vi "AppLauncher.vi"() -> ()   [LabVIEW 2016, in "Instrument.SR7270.lvclass"]
uses:
  Instrument.SR7270.lvclass
  <vilib>/JKI/JKI SMO/SMO/SMO.lvclass
  <vilib>/JKI/JKI SMO/SMO/Typedefs/SMOState --Enum.ctl
  <vilib>/JKI/JKI SMO/SMO.UI/SMO.UI.lvclass
  SR7270 UI/SR7270 UI.lvclass
  C:/user/patrick/hg/levylab_inst/lvsrc/SMOs/Instrument/Instrument.lvclass
  C:/Program Files (x86)/National Instruments/LabVIEW 2016/vi.lib/JKI/JKI SMO/SMO/SMO.lvclass
  C:/Program Files (x86)/National Instruments/LabVIEW 2016/vi.lib/JKI/JKI SMO/SMO.UI/SMO.UI.lvclass
  <vilib>/Utility/sysdir.llb/System Directory Type.ctl
panel:
  out "UI SMO State":T1
  out "SMO State":T1
  out "error out":errorcluster
  in  "Stop":bool
  # "Instrument.SR7270 SMO Launcher"
  # "For instructions on how to use the JKI State Machine Objects, examples and video tutorials, visit:\nhttp://jki.net/state-machine-objects/\n\nJKI State Machine Objects™\nhttp://jki.net/state-machine-objects/\nCopyright (C) 2005-2015, JKI <info@jki.net>\nALL RIGHTS RESERVED"
  # "Starting SR7270 SMO..."
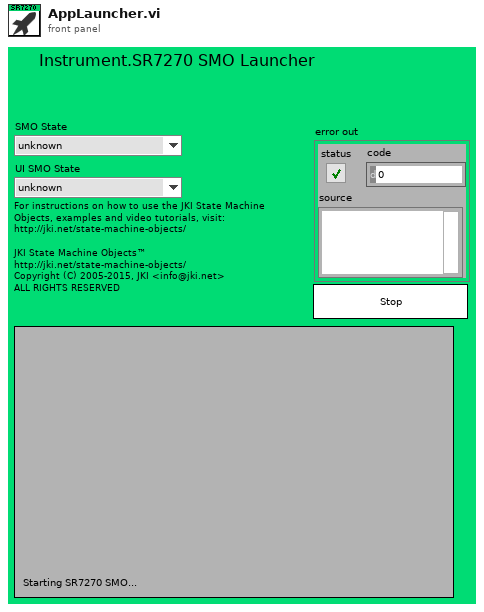
[diagram p1: front panel]
types:
  T1 = typedef "SMO.lvclass/SMOState --Enum.ctl" = enum16{"unknown", "Created", "Started", "Stopped"}
  T2 = typedef "System Directory Type.ctl" = i32
  T3 = typedef "SMO.lvclass/Public Events.ctl" = cluster{"Error":refnum<user-event>, "State":refnum<user-event>, "Reserve State":refnum<user-event>}
  T4 = cluster{"Event Registration Refnum":refnum<event-registration>, "Event Registration Refnum":refnum<event-registration>}
  T5 = enum32{"Invalid", "Standard", "Closed", "Hidden", "Minimized", "Maximized"}
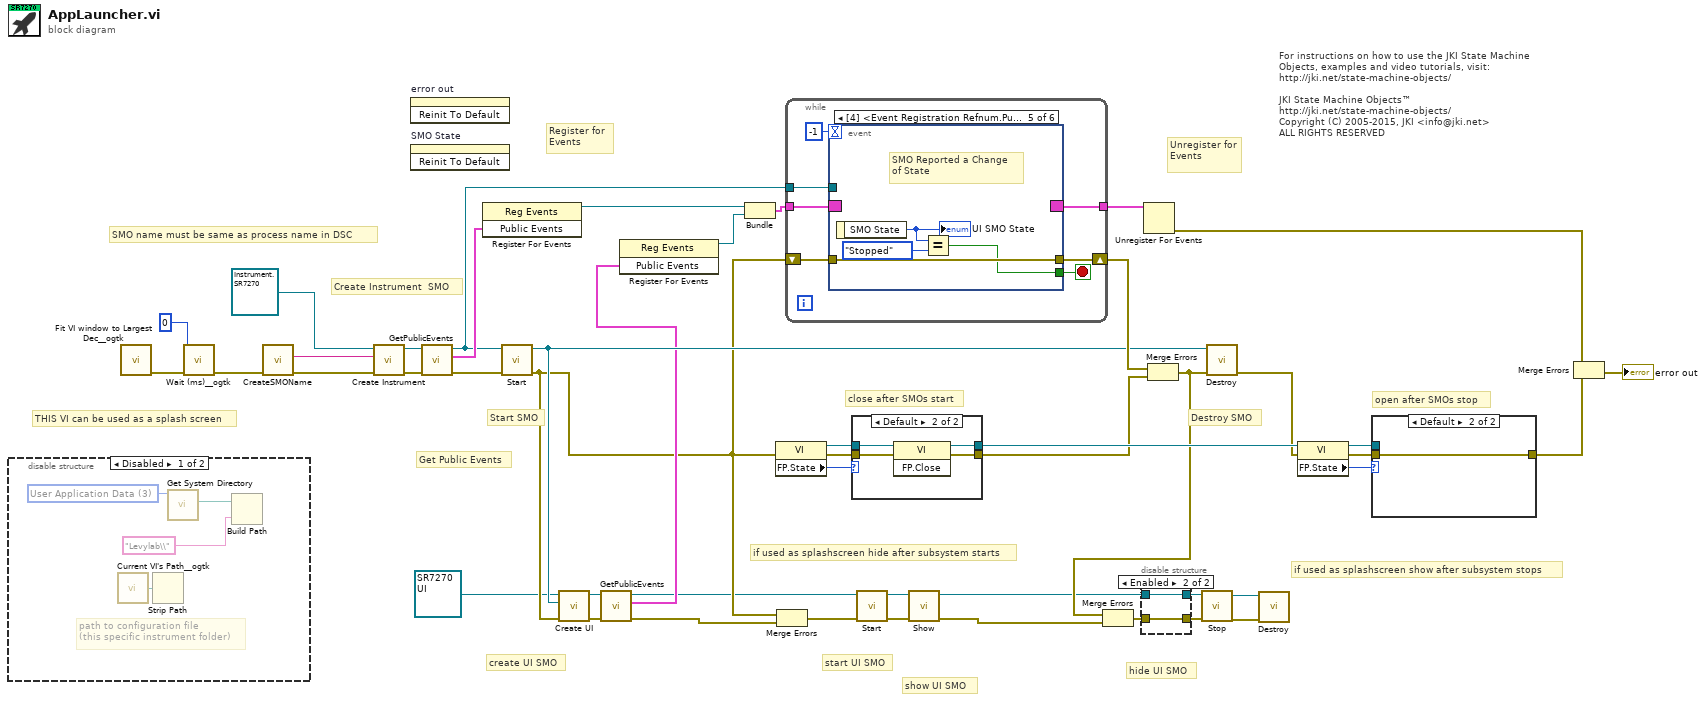
[diagram p0: block diagram]
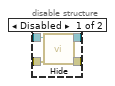
[diagram p3: hidden frame]
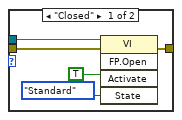
[diagram p4: hidden frame]
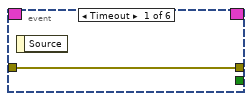
[diagram p6: hidden frame]
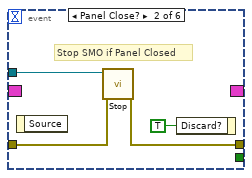
[diagram p7: hidden frame]
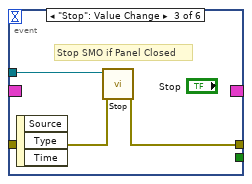
[diagram p8: hidden frame]
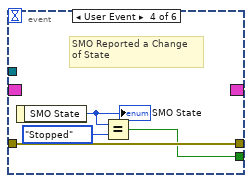
[diagram p9: hidden frame]
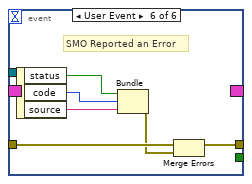
[diagram p10: hidden frame]
diagram:
  # "open after SMOs stop"
  # "close after SMOs start"
  # "hide UI SMO"
  # "show UI SMO"
  # "start UI SMO"
  # "create UI SMO"
  # "if used as splashscreen show after subsystem stops"
  # "if used as splashscreen hide after subsystem starts"
  # "THIS VI can be used as a splash screen"
  # "SMO name must be same as process name in DSC"
  # "Get Public Events"
  # "Start SMO"
  # "Destroy SMO"
  # "Create Instrument  SMO"
  # "Unregister for Events"
  # "Register for Events"
  # "For instructions on how to use the JKI State Machine Objects, examples and video tutorials, visit:\nhttp://jki.net/state-machine-objects/\n\nJKI State Machine Objects™\nhttp://jki.net/state-machine-objects/\nCopyright (C) 2005-2015, JKI <info@jki.net>\nALL RIGHTS RESERVED"
  n1 = disable-structure shown="Disabled" {
    frame Disabled {
      w50 = T2 3 items=["User Home"=0, "User Desktop"=1, "User Documents"=2, "User Application Data"=3, "User Preferences"=4, "User Temporary"=5, "Public Documents"=6, "Public Application Data"=7, "Public Preferences"=8, "Public Cache"=13, "System Core Libraries"=9, "System Installed Libraries"=10, "Application Files"=11, "Boot Volume Root"=12] ("system directory type")
      # "path to configuration file\n(this specific instrument folder)"
      n2 = call <userlib>:"Current VI's Path__ogtk.vi"() -> ("Current VI's Path (+ Relative)"=w51:path)  [unwired: 1 in]
      n3 = Strip Path(path=w51) -> ()  [unwired: 2 out]
      n4 = call <vilib>:"Get System Directory.vi"("system directory type"=w50) -> ("system directory"=w49:path)  [unwired: 10 in]
      n5 = Build Path(base path=w49, name or relative path="Levylab\\") -> ()  [unwired: 1 out]
    }
    frame Enabled {
    }
  }
  n6 = call <userlib>:"Fit VI window to Largest Dec__ogtk.vi"() -> ("error out"=w34:errorcluster)  [unwired: 6 in, 1 out]
  n7 = call <userlib>:"Wait (ms)__ogtk.vi"("error in (no error)"=w34, "milliseconds to wait"=u32 0) -> ("error out"=w3:errorcluster)  [unwired: 8 in, 1 out]
  n8 = call "CreateSMOName.vi"("error in (no error)"=w3) -> ("error out"=w1:errorcluster, "Name"=w2:string)  [unwired: 9 in]
  n9 = call-dynamic "Create Instrument.vi"("error in (no error)"=w1, "Subsystem Name"=w2, "Instrument in"=refnum<class "Instrument.SR7270.lvclass"> refnum ("Instrument.SR7270.lvclass")) -> ("error out"=w41:errorcluster, "Instrument out"=w42:refnum<class "Instrument.SR7270.lvclass">)  [unwired: 7 in]
  n10 = invoke on="error out" class="Clust (strict)" method="Reinit To Default"() -> ()  [unwired: 3 in, 3 out]
  n11 = invoke on="SMO State" class="Enum (strict)" method="Reinit To Default"() -> ()  [unwired: 3 in, 3 out]
  n12 = call <vilib>:"GetPublicEvents.vi"("error in (no error)"=w41, "SMO"=w42) -> ("error out"=w40:errorcluster, "Public Events"=w44:T3, "SMO out"=w43:refnum<class "Instrument.SR7270.lvclass">)  [unwired: 7 in]
  n13 = register-events(w44) -> (reference out=w33:refnum<event-registration>)  [unwired: 2 in, 1 out]
  n14 = call <vilib>:"Start.vi"("error in (no error)"=w40, "SMO"=w43) -> ("error out"=w26:errorcluster, "SMO out"=w31:refnum<class "Instrument.SR7270.lvclass">)  [unwired: 8 in]
  n15 = call "Create UI.vi"("error in (no error)"=w26, "Instrument in"=w31, "SR7270 UI in"=refnum<class "SR7270 UI.lvclass"> refnum ("SR7220 UI.lvclass")) -> ("error out"=w29:errorcluster, "SR7270 UI out"=w28:refnum<class "SR7270 UI.lvclass">)  [unwired: 7 in]
  n16 = call <vilib>:"GetPublicEvents.vi"("error in (no error)"=w29, "SMO"=w28) -> ("error out"=w20:errorcluster, "Public Events"=w27:T3, "SMO out"=w21:refnum<class "SR7270 UI.lvclass">)  [unwired: 7 in]
  n17 = register-events(w27) -> (reference out=w30:refnum<event-registration>)  [unwired: 2 in, 1 out]
  n18 = Bundle("Event Registration Refnum"=w33, "Event Registration Refnum"=w30) -> (w32:T4)  [unwired: 1 in]
  n19 = property class="VI"(error in=w26) -> (reference out=w9:refnum<vi>, error out=w10:errorcluster, "FP.State"=w8:T5)  [unwired: 1 in]
  n20 = Merge Errors(w26, w20) -> (w25:errorcluster)
  n21 = while {
    shift-right: [w57] -> w39
    shift-left: w26 -> [w56]
    tunnel: w32 -> [w55]
    tunnel: [w54] -> w47
    tunnel: w43 -> [w53]
    stop <- w58 stop-if-true
    n22 = event shown="[4] <Event Registration Refnum.Public Events.State>: User Event" {
      selector: w55 -> [_ _ _ _ _ _]
      dyn-events: [_ _ _ _ _ _] -> w54
      timeout: -1 -> [_ _ _ _ _ _]
      tunnel: [_ _ _ w67 w71 _] -> w58
      tunnel: w53 -> [_ w63 w66 _ _ _]
      tunnel: [w59 w62 w65 w70 w74 w78] -> w57
      tunnel: w56 -> [w59 w61 w64 w70 w74 w76]
      event Timeout {
        n23 = event-data() -> ()  [unwired: 1 in, 1 out]
      }
      event Panel Close? {
        # "Stop SMO if Panel Closed"
        n24 = event-data() -> ()  [unwired: 1 in, 1 out]
        n25 = call <vilib>:"Stop.vi"("error in (no error)"=w61, "SMO"=w63) -> ("error out"=w62:errorcluster)  [unwired: 8 in, 1 out]
        n26 = event-data("Discard?"=TRUE ("OK")) -> ()  [unwired: 1 in, 1 out]
      }
      event "Stop": Value Change {
        # "Stop SMO if Panel Closed"
        n27 = event-data() -> ()  [unwired: 1 in, 3 out]
        n28 = call <vilib>:"Stop.vi"("error in (no error)"=w64, "SMO"=w66) -> ("error out"=w65:errorcluster)  [unwired: 8 in, 1 out]
      }
      event User Event {
        # "SMO Reported a Change\nof State"
        n29 = event-data() -> ("SMO State"=w69:T1)  [unwired: 1 in]
        "SMO State" <- w69
        n30 = Equal?(x=w69, y=SMOState_--Enum."Stopped") -> (x = y?=w67:bool)
      }
      event User Event {
        # "SMO Reported a Change\nof State"
        n31 = event-data() -> ("SMO State"=w73:T1)  [unwired: 1 in]
        "UI SMO State" <- w73
        n32 = Equal?(x=w73, y=SMOState_--Enum."Stopped") -> (x = y?=w71:bool)
      }
      event User Event {
        # "SMO Reported an Error"
        n33 = event-data() -> ("status"=w77:bool, "code"=w80:i32, "source"=w79:string)  [unwired: 1 in]
        n34 = Bundle("status"=w77, "code"=w80, "source"=w79) -> (w75:errorcluster)  [unwired: 1 in]
        n35 = Merge Errors(w76, w75) -> (w78:errorcluster)
      }
    }
  }
  n36 = case shown="Default" w8 {
    tunnel: [w82 w86] -> w35
    tunnel: w10 -> [w82 w85]
    tunnel: w9 -> [w81 w84]
    tunnel: [w81 w83] -> w38
    frame "Invalid", "Closed" {
    }
    frame Default {
      n37 = invoke class="VI" method="FP.Close"(reference=w84, error in=w85) -> (reference out=w83:refnum<vi>, error out=w86:errorcluster)  [unwired: 1 in, 1 out]
    }
  }
  n38 = call <vilib>:"Start.vi"("error in (no error)"=w25, "SMO"=w21) -> ("error out"=w19:errorcluster, "SMO out"=w18:refnum<class "SR7270 UI.lvclass">)  [unwired: 8 in]
  n39 = call <vilib>:"Show.vi"("error in (no error)"=w19, "SMO.UI"=w18) -> ("error out"=w17:errorcluster, "SMO.UI out"=w13:refnum<class "SR7270 UI.lvclass">)  [unwired: 8 in]
  n40 = Unregister For Events(event registration refnum=w47) -> (error out=w46:errorcluster)  [unwired: 1 in]
  n41 = Merge Errors(w39, w35) -> (w22:errorcluster)
  n42 = Merge Errors(w22, w17) -> (w14:errorcluster)
  n43 = disable-structure shown="Enabled" {
    disable-tunnel: [w90 w91] -> w16
    disable-tunnel: [w89 w92] -> w15
    disable-tunnel: w14 -> [w88 w91]
    disable-tunnel: w13 -> [w87 w92]
    frame Disabled {
      n44 = call <vilib>:"Hide.vi"("error in (no error)"=w88, "SMO.UI"=w87) -> ("error out"=w90:errorcluster, "SMO.UI out"=w89:refnum<class "SR7270 UI.lvclass">)  [unwired: 8 in]
    }
    frame Enabled {
    }
  }
  n45 = call <vilib>:"Stop.vi"("error in (no error)"=w16, "SMO"=w15) -> ("error out"=w24:errorcluster, "SMO out"=w23:refnum<class "SR7270 UI.lvclass">)  [unwired: 8 in]
  n46 = call <vilib>:"Destroy.vi"("error in (no error)"=w22, "SMO"=w31) -> ("error out"=w37:errorcluster)  [unwired: 9 in]
  n47 = call <vilib>:"Destroy.vi"("error in (no error)"=w24, "SMO"=w23) -> ()  [unwired: 9 in, 1 out]
  n48 = property class="VI"(reference=w38, error in=w37) -> (reference out=w6:refnum<vi>, error out=w7:errorcluster, "FP.State"=w5:T5)
  n49 = case shown="Default" w5 {
    tunnel: [w95 w98] -> w36
    tunnel: w7 -> [w94 w98]
    tunnel: w6 -> [w93 _]
    frame "Closed" {
      n50 = invoke class="VI" method="FP.Open"(reference=w93, error in=w94, "Activate"=TRUE, "State"=T5."Standard") -> (error out=w95:errorcluster)  [unwired: 1 in, 4 out]
    }
    frame Default {
    }
  }
  n51 = Merge Errors(w46, w36) -> (→"error out":errorcluster)
